vi "Simulation Kobuki Open.vi"(8 "error in (no error)":errorcluster) -> (0 "error out":errorcluster, 2 "initial position":sgl[](array[numeric]), 3 "simulator":T1={"configuration"={"maxTime"=5.0, "enableVisualization"=TRUE, "statechart"=path "iRobot Navigation State Machine.vi", "environment"=path "simulation configuration.ini", "record"=path "Simulation Record.xml", "autograde?"=TRUE, "interactive?"=FALSE, "feedback mode"=enum."debug navigation"}, "Bump Sensors"=[], "Distance Sensors"=[], "Accelerometer"=refnum, "Wall Sensor"=refnum, "Statechart\ndisplay"=refnum, "Body"=refnum, "Left Motor"=refnum, "Right Motor"=refnum, "first step?"=FALSE})   [LabVIEW 2014]
doc: "Begins a simulation of the Cal Climber."
uses:
  Simulator.ctl
  <instrlib>/DC Motor Controller/HAIOL/DC Motor Controller.lvclass
  CyberSim interface/Simulation Configuration.ctl
  autograder/feedbackMode.ctl
  <vilib>/Robotics/Simulator/Engine/ctl/DeviceID.ctl
  <vilib>/Robotics/Simulator/Interface/Simulator References/Get Sensor Reference.vi
  <vilib>/Robotics/Simulator/Interface/Simulator References/Get Robot Body Reference.vi
  <vilib>/robotics/Simulator/NI_Robotics_Simulator.lvlib
  <resource>/objmgr/LVODE.rc
  <instrlib>/DC Motor Controller/HAIOL/Simulator/DC Motor Controller Simulator.lvclass
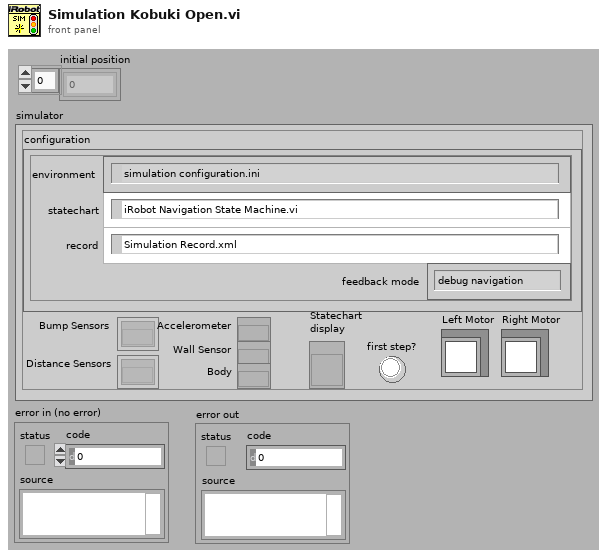
[diagram p1: front panel]
types:
  T1 = typedef "Simulator.ctl" = cluster{"configuration":T2, "Bump Sensors":refnum<k20>[], "Distance Sensors":refnum<k20>[], "Accelerometer":refnum<k20>, "Wall Sensor":refnum<k20>, "Statechart\ndisplay":refnum<vi>, "Body":refnum<k20>, "Left Motor":refnum<class "DC Motor Controller.lvclass">, "Right Motor":refnum<class "DC Motor Controller.lvclass">, "first step?":bool}
  T2 = typedef "Simulation Configuration.ctl" = cluster{"maxTime":sgl, "enableVisualization":bool, "statechart":path, "environment":path, "record":path, "autograde?":bool, "interactive?":bool, "feedback mode":T3}
  T3 = typedef "feedbackMode.ctl" = enum32{"debug navigation", "debug hill climb", "autograde navigation", "autograde hill climb"}
  T4 = typedef "NI_Robotics_Simulator.lvlib/DeviceID.ctl" = cluster{"robot ID":string, "sensor/actuator ID":string}
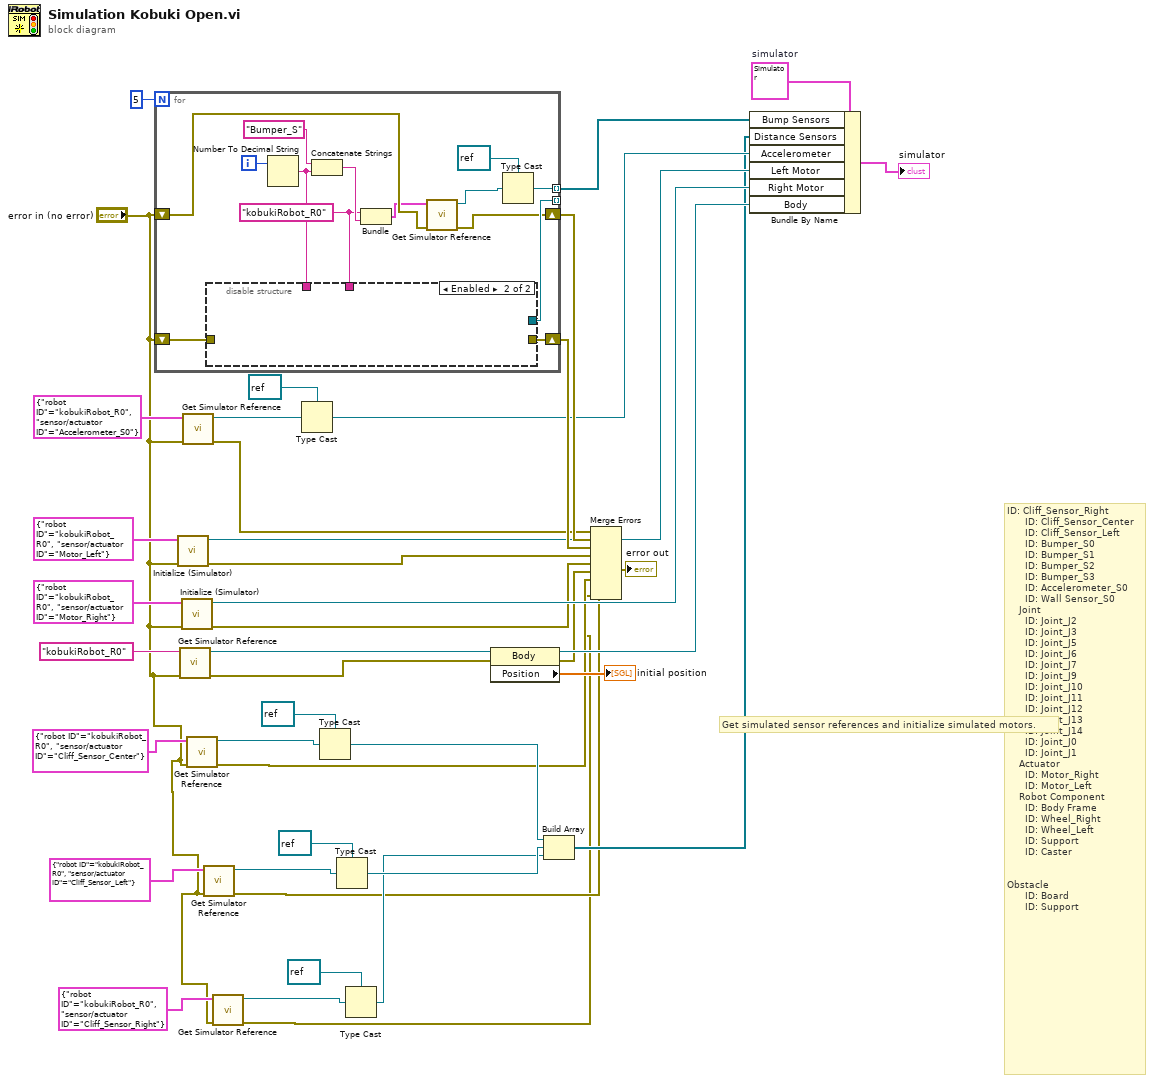
[diagram p0: block diagram]
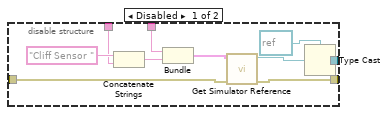
[diagram p2: hidden frame]
diagram:
  w36 = T1 {"configuration"={"maxTime"=0.0, "enableVisualization"=FALSE, "statechart"=path "", "environment"=path "", "record"=path "", "autograde?"=FALSE, "interactive?"=FALSE, "feedback mode"=enum."debug navigation"}, "Bump Sensors"=[], "Distance Sensors"=[], "Accelerometer"=refnum, "Wall Sensor"=refnum, "Statechart\ndisplay"=refnum, "Body"=refnum, "Left Motor"=refnum, "Right Motor"=refnum, "first step?"=FALSE}  # simulator
  # "ID: Cliff_Sensor_Right\n\t\t\t\t\t\tID: Cliff_Sensor_Center\n\t\t\t\t\t\tID: Cliff_Sensor_Left\n\t\t\t\t\t\tID: Bumper_S0\n\t\t\t\t\t\tID: Bumper_S1\n\t\t\t\t\t\tID: Bumper_S2\n\t\t\t\t\t\tID: Bumper_S3\n\t\t\t\t\t\tID: Accelerometer_S0\n\t\t\t\t\t\tID: Wall Sensor_S0\n\t\t\t\tJoint\n\t\t\t\t\t\tID: Joint_J2\n\t\t\t\t\t\tID: Joint_J3\n\t\t\t\t\t\tID: Joint_J5\n\t\t\t\t\t\tID: Joint_J6\n\t\t\t\t\t\tID: Joint_J7\n\t\t\t\t\t\tID: Joint_J9\n\t\t\t\t\t\tID: Joint_J10\n\t\t\t\t\t\tID: Joint_J11\n\t\t\t\t\t\tID: Joint_J12\n\t\t\t\t\t\tID: Joint_J13\n\t\t\t\t\t\tID: Joint_J14\n\t\t\t\t\t\tID: Joint_J0\n\t\t\t\t\t\tID: Joint_J1\n\t\t\t\tActuator\n\t\t\t\t\t\tID: Motor_Right\n\t\t\t\t\t\tID: Motor_Left\n\t\t\t\tRobot Component\n\t\t\t\t\t\tID: Body Frame\n\t\t\t\t\t\tID: Wheel_Right\n\t\t\t\t\t\tID: Wheel_Left\n\t\t\t\t\t\tID: Support\n\t\t\t\t\t\tID: Caster\n\n\nObstacle\n\t\t\t\t\t\tID: Board\n\t\t\t\t\t\tID: Support"
  # "Get simulated sensor references and initialize simulated motors."
  n1 = for {
    N: 5 -> [_]
    tunnel: [w54] -> _ mode=indexing
    tunnel: [w49] -> w37 mode=indexing
    shift-right: [w44] -> w38
    shift-left: "error in (no error)" -> [w47]
    shift-right: [w42] -> w39
    shift-left: "error in (no error)" -> [w43]
    i -> [w55]
    w48 = "kobukiRobot_R0" ("Robot ID")
    n2 = Number To Decimal String(number=w55) -> (decimal integer string=w52:string)  [unwired: 1 in]
    n3 = disable-structure shown="Enabled" {
      disable-tunnel: [w63 _] -> w54
      disable-tunnel: w52 -> [w61 _]
      disable-tunnel: w48 -> [w60 _]
      disable-tunnel: w43 -> [w58 _]
      disable-tunnel: [w57 _] -> w42
      frame Disabled {
        n4 = Concatenate Strings("Cliff Sensor " ("Device Label"), w61) -> (w64:string)
        n5 = Bundle("Robot ID"=w60, w64) -> (w59:cluster{"Robot ID":string, string})  [unwired: 1 in]
        n6 = call-poly <vilib>:"Get Simulator Reference.vi"("error in (no error)"=w58, "device ID"=w59) -> ("error out"=w57:errorcluster, "sensor ref"=w56:refnum<k20>)  [unwired: 8 in]
        n7 = Type Cast(type=refnum<k20> refnum ("DistanceSensor Out"), x=w56) -> (*(type *) &x=w63:refnum<k20>)
      }
      frame Enabled {
      }
    }
    n8 = Concatenate Strings("Bumper_S" ("Device Label"), w52) -> (w51:string)
    n9 = Bundle("Robot ID"=w48, w51) -> (w46:cluster{"Robot ID":string, string})  [unwired: 1 in]
    n10 = call-poly <vilib>:"Get Simulator Reference.vi"("error in (no error)"=w47, "device ID"=w46) -> ("error out"=w44:errorcluster, "sensor ref"=w45:refnum<k20>)  [unwired: 8 in]
    n11 = Type Cast(type=refnum<k20> refnum ("DistanceSensor Out"), x=w45) -> (*(type *) &x=w49:refnum<k20>)
  }
  n12 = call <instrlib>:"Initialize (Simulator).vi"("error in (no error)"="error in (no error)", "Device ID"=T4 {"robot ID"="kobukiRobot_R0", "sensor/actuator ID"="Motor_Left"}) -> ("error out"=w26:errorcluster, "DC Motor Controller out"=w27:refnum<class "DC Motor Controller.lvclass">)  [unwired: 8 in]
  n13 = call-poly <vilib>:"Get Simulator Reference.vi"("error in (no error)"="error in (no error)", "robot ID"="kobukiRobot_R0" ("Robot ID")) -> ("error out"=w20:errorcluster, "robot body ref"=w21:refnum<k20>)  [unwired: 8 in]
  n14 = call <instrlib>:"Initialize (Simulator).vi"("error in (no error)"="error in (no error)", "Device ID"=T4 {"robot ID"="kobukiRobot_R0", "sensor/actuator ID"="Motor_Right"}) -> ("error out"=w23:errorcluster, "DC Motor Controller out"=w24:refnum<class "DC Motor Controller.lvclass">)  [unwired: 8 in]
  n15 = call-poly <vilib>:"Get Simulator Reference.vi"("error in (no error)"="error in (no error)", "device ID"=T4 {"robot ID"="kobukiRobot_R0", "sensor/actuator ID"="Accelerometer_S0"} ("Device ID")) -> ("error out"=w19:errorcluster, "sensor ref"=w29:refnum<k20>)  [unwired: 8 in]
  n16 = call-poly <vilib>:"Get Simulator Reference.vi"("error in (no error)"="error in (no error)", "device ID"=T4 {"robot ID"="kobukiRobot_R0", "sensor/actuator ID"="Cliff_Sensor_Center"} ("Device ID")) -> ("error out"=w3:errorcluster, "sensor ref"=w15:refnum<k20>)  [unwired: 8 in]
  n17 = call-poly <vilib>:"Get Simulator Reference.vi"("error in (no error)"="error in (no error)", "device ID"=T4 {"robot ID"="kobukiRobot_R0", "sensor/actuator ID"="Cliff_Sensor_Left"} ("Device ID")) -> ("error out"=w2:errorcluster, "sensor ref"=w14:refnum<k20>)  [unwired: 8 in]
  n18 = call-poly <vilib>:"Get Simulator Reference.vi"("error in (no error)"="error in (no error)", "device ID"=T4 {"robot ID"="kobukiRobot_R0", "sensor/actuator ID"="Cliff_Sensor_Right"} ("Device ID")) -> ("error out"=w1:errorcluster, "sensor ref"=w9:refnum<k20>)  [unwired: 8 in]
  n19 = Type Cast(type=refnum<k20> refnum ("DistanceSensor Out"), x=w29) -> (*(type *) &x=w35:refnum<k20>)
  n20 = Type Cast(type=refnum<k20> refnum ("DistanceSensor Out"), x=w15) -> (*(type *) &x=w7:refnum<k20>)
  n21 = Type Cast(type=refnum<k20> refnum ("DistanceSensor Out"), x=w14) -> (*(type *) &x=w6:refnum<k20>)
  n22 = Type Cast(type=refnum<k20> refnum ("DistanceSensor Out"), x=w9) -> (*(type *) &x=w5:refnum<k20>)
  n23 = property class="Body"(reference=w21, error in=w20) -> (reference out=w34:refnum<k20>, error out=w18:errorcluster, "Position"=→"initial position":sgl[])
  n24 = Build Array(w7, w6, w5) -> (w4:refnum<k20>[])
  n25 = Merge Errors(w19, w38, w39, w26, w23, w18, w3, w2, w1) -> (→"error out":errorcluster)
  n26 = Bundle By Name(cluster=w36, "Bump Sensors"=w37, "Distance Sensors"=w4, "Accelerometer"=w35, "Left Motor"=w27, "Right Motor"=w24, "Body"=w34) -> (→"simulator":T1)
